vi "UsrProfiles-Check profile changed.vi"(8 "error in (no error)":errorcluster) -> (0 "error out":errorcluster, 3 "Profile changed":bool)   [LabVIEW 2017]
uses:
  Global Variables/General Globals.vi
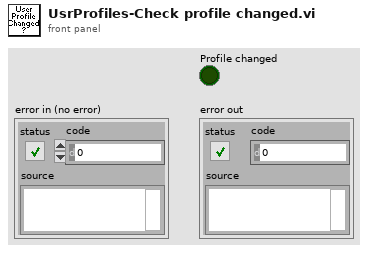
[diagram p1: front panel]
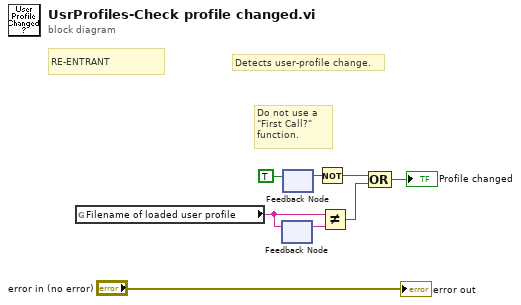
[diagram p0: block diagram]
diagram:
  # "Do not use a \"First Call?\" function."
  # "Detects user-profile change."
  # "RE-ENTRANT"
  n1 = global read "General Globals.vi" "Filename of loaded user profile"() -> (w8:string)
  n2 = feedback #1() -> (w7:string)  [unwired: 1 in]
  n3 = feedback-in #1(w8) -> ()
  n4 = feedback #2() -> (w4:bool)  [unwired: 1 in]
  n5 = feedback-in #2(TRUE) -> ()
  n6 = Not(x=w4) -> (.not. x?=w3:bool)
  n7 = Not Equal?(x=w8, y=w7) -> (x != y?=w2:bool)
  n8 = Compound Arithmetic op=OR(w3, w2) -> (→"Profile changed":bool)
  "error out" <- "error in (no error)"
